vi "Set XScale.vi"(8 "error in (no error)":errorcluster caption="entrée d'erreur (pas d'erreur)", 10 "Section":string="UV-VIS", 11 "Detector en entrée":refnum<class "Detector.lvclass">) -> (0 "error out":errorcluster caption="sortie d'erreur", 3 "Detector en sortie":refnum<class "Detector.lvclass">)   [LabVIEW 2015, in "Detector.lvclass"]
uses:
  Detector.lvclass
  GeneralFunctionality/GeneralFunctionality.lvclass/GeneralFunctionality.ctl
  Detector.lvclass/Detector.ctl
  dependecies/globalVarII.vi
  <vilib>/Utility/file.llb/Read Delimited Spreadsheet (DBL).vi
  Config/Config.lvclass
  GeneralFunctionality/GeneralFunctionality.lvclass
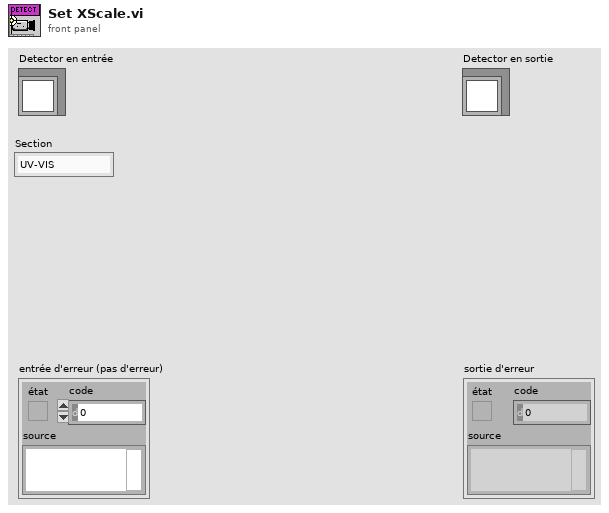
[diagram p1: front panel]
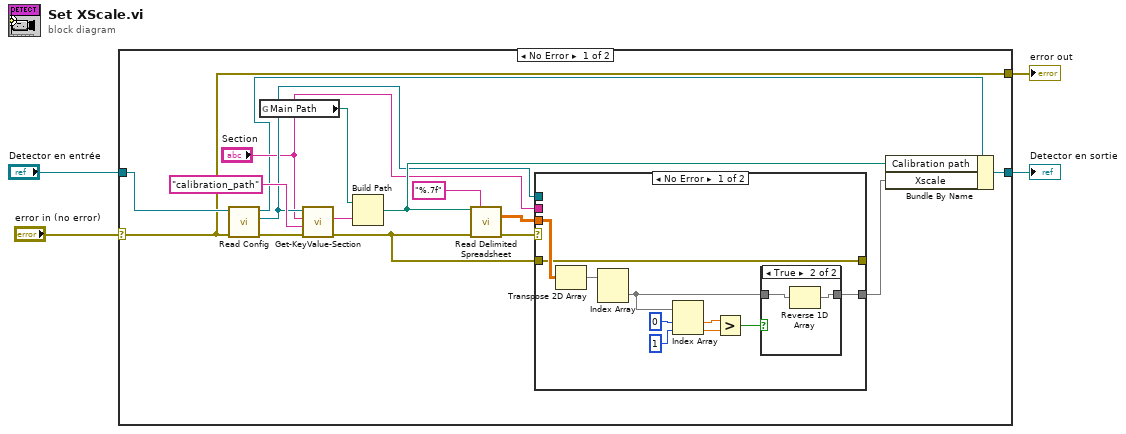
[diagram p0: block diagram]
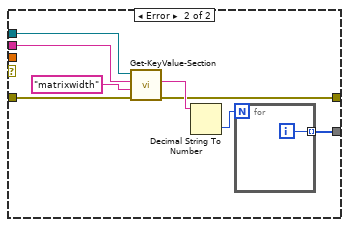
[diagram p3: hidden frame]
diagram:
  n1 = case shown="No Error" "error in (no error)" {
    selector: "error in (no error)" -> [w18 w44]
    tunnel: [w18 w44] -> w3
    tunnel: [w20 w43] -> w1
    tunnel: "Detector en entrée" -> [w19 w43]
    frame No Error {
      n2 = call "Read Config.vi"("error in (no error)"=w18, "GeneralFunctionality en entrée"=w19) -> ("error out"=w17:errorcluster, "Config.lvclass"=w10:refnum<class "Config.lvclass">, "GeneralFunctionality en sortie"=w5:refnum<class "Detector.lvclass">)  [unwired: 7 in]
      n3 = global read "globalVarII.vi" "Main Path"() -> (w14:path)
      n4 = call-dynamic "Get-KeyValue-Section.vi"("error in (no error)"=w17, "Key"="calibration_path", "Section"="Section", "Config in"=w10) -> ("error out"=w8:errorcluster, "Value"=w15:string)  [unwired: 5 in, 1 out]
      n5 = Build Path(base path=w14, name or relative path=w15) -> (appended path=w13:path)
      n6 = call-poly <vilib>:"Read Delimited Spreadsheet.vi"("file path (dialog if empty)"=w13, "format (%.3f)"="%.7f", "error in (no error)"=w8) -> ("all rows"=w11:dbl[][], "error out"=w12:errorcluster)  [unwired: 7 in, 4 out]
      n7 = case shown="No Error" w12 {
        tunnel: w11 -> [w30 _]
        tunnel: [w28 w35] -> _
        tunnel: [w21 w36] -> w6
        tunnel: w10 -> [_ w41]
        tunnel: "Section" -> [_ w40]
        tunnel: w8 -> [w28 w38]
        frame No Error {
          n8 = Transpose 2D Array(2D array=w30) -> (transposed array=w29:dbl[][])
          n9 = Index Array(array=w29) -> (element=w22:dbl[])  [unwired: 2 in]
          n10 = Index Array(array=w22, index #1=0 ("index"), index #2=1 ("index")) -> (element #1=w25:dbl, element #2=w26:dbl)
          n11 = Greater?(x=w25, y=w26) -> (0:w27:bool)
          n12 = case shown="True" w27 {
            tunnel: w22 -> [w31 w33]
            tunnel: [w31 w32] -> w21
            frame False {
            }
            frame True {
              n13 = Reverse 1D Array(array=w33) -> (reversed array=w32:dbl[])
            }
          }
        }
        frame Error {
          n14 = call-dynamic "Get-KeyValue-Section.vi"("error in (no error)"=w38, "Key"="matrixwidth", "Section"=w40, "Config in"=w41) -> ("error out"=w35:errorcluster, "Value"=w37:string)  [unwired: 5 in, 1 out]
          n15 = Decimal String To Number(string=w37) -> (number=w34:i32)  [unwired: 2 in, 1 out]
          n16 = for {
            N: w34 -> [_]
            tunnel: [w42] -> w36 mode=indexing
            i -> [w42]
          }
        }
      }
      n17 = Bundle By Name(cluster=w5, "Calibration path"=w13, "Xscale"=w6) -> (w20:refnum<class "Detector.lvclass">)
    }
    frame Error {
    }
  }
  "error out" <- w3
  "Detector en sortie" <- w1
